vi "Get App Version.vi"() -> (0 "runtime":bool, 1 "App. Version Number":string)   [LabVIEW 2020, in "dsdll.lvlib"]
doc: "Returns application version number for compiled exe file. In the case of developement or other, returns describing text."
uses:
  dsdll.lvlib
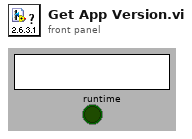
[diagram p1: front panel]
types:
  T1 = enum32{"invalid app kind", "Development System", "Run Time System", "Student Edition", "Embedded LabVIEW", "Evaluation", "Custom"}
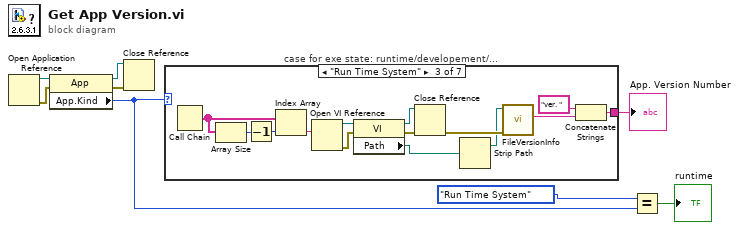
[diagram p0: block diagram]
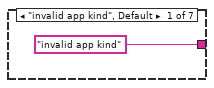
[diagram p2: hidden frame]
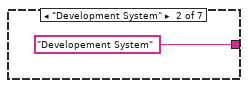
[diagram p3: hidden frame]
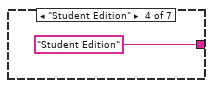
[diagram p4: hidden frame]
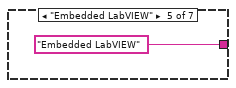
[diagram p5: hidden frame]
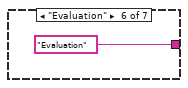
[diagram p6: hidden frame]
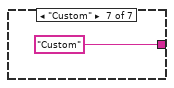
[diagram p7: hidden frame]
diagram:
  n1 = Open Application Reference() -> (0:w3:errorcluster, 3:w8:refnum<vi>)  [unwired: 4 in]
  n2 = property class="App"(reference=w8, error in=w3) -> (reference out=w1:refnum<vi>, error out=w2:errorcluster, "App.Kind"=w5:T1)
  n3 = Close Reference(reference=w1, error in (no error)=w2) -> ()  [unwired: 1 out]
  n4 = case "case for exe state: runtime/developement/..." shown="\"Run Time System\"" w5 {
    tunnel: ["invalid app kind" "Developement System" w22 "Student Edition" "Embedded LabVIEW" "Evaluation" "Custom"] -> w7
    frame "invalid app kind", Default {
    }
    frame "Development System" {
    }
    frame "Run Time System" {
      n5 = Call Chain() -> (call chain=w18:string[])
      n6 = Array Size(array=w18) -> (size(s)=w19:i32)
      n7 = Decrement(x=w19) -> (x-1=w17:i32)
      n8 = Index Array(array=w18, index=w17) -> (element=w16:string)
      n9 = Open VI Reference(vi path=w16) -> (vi reference=w20:refnum<vi>, error out=w21:errorcluster)  [unwired: 5 in]
      n10 = property class="VI"(reference=w20, error in=w21) -> (reference out=w14:refnum<vi>, error out=w15:errorcluster, "Path"=w12:path)
      n11 = Close Reference(reference=w14, error in (no error)=w15) -> (error out=w13:errorcluster)
      n12 = Strip Path(path=w12) -> (stripped path=w11:path)  [unwired: 1 out]
      n13 = call <vilib>:"FileVersionInfo.vi"("error in (no error)"=w13, "Application Path in"=w11) -> ("File Version Info"=w23:string)  [unwired: 6 in, 3 out]
      n14 = Concatenate Strings("ver. " ("string"), w23) -> (w22:string)
    }
    frame "Student Edition" {
    }
    frame "Embedded LabVIEW" {
    }
    frame "Evaluation" {
    }
    frame "Custom" {
    }
  }
  "App. Version Number" <- w7
  n15 = Equal?(x=T1."Run Time System" ("Application:Kind"), y=w5) -> (x = y?=→"runtime":bool)
